vi "Get Status_All Records One.vi"(7 "Timeout (s)":dbl=5.0 caption="Time Target (s)", 8 "error in":errorcluster, 11 "FPGA VI Reference In":refnum<k20>) -> (0 "error out":errorcluster, 2 "Records Done":u32, 3 "FPGA VI Reference Out":refnum<k20>)   [LabVIEW 2011]
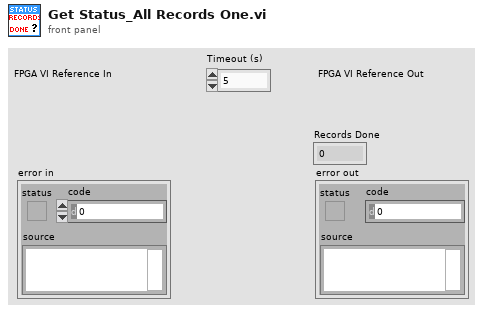
[diagram p1: front panel]
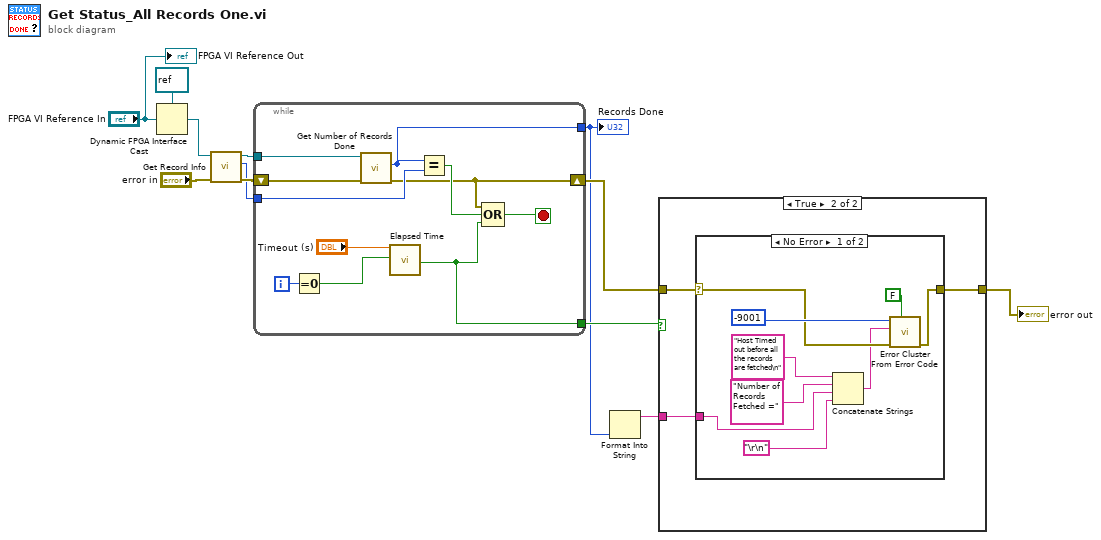
[diagram p0: block diagram]
diagram:
  n1 = Dynamic FPGA Interface Cast(Session In=refnum<k20> refnum ("Type"), Type="FPGA VI Reference In") -> (Session Out=w8:refnum<k20>)
  n2 = call <userlib>:"Get Record Info.vi"("error in"="error in", "FPGA VI Reference In"=w8) -> ("error out"=w12:errorcluster, "Records to Acquire"=w10:u32, "FPGA VI Reference Out"=w11:refnum<k20>)  [unwired: 5 in, 2 out]
  n3 = while {
    tunnel: w11 -> [w21]
    shift-right: [w16] -> w4
    shift-left: w12 -> [w23]
    tunnel: w10 -> [w22]
    tunnel: [w20] -> w2
    tunnel: [w15] -> w5
    i -> [w14]
    stop <- w17 stop-if-true
    n4 = Equal To 0?(x=w14) -> (x = 0?=w13:bool)
    n5 = call <userlib>:"Get Number of Records Done.vi"("error in"=w23, "FPGA VI Reference In"=w21) -> ("error out"=w16:errorcluster, "Records Done"=w20:u32)  [unwired: 7 in, 1 out]
    n6 = call "Elapsed Time"("Time Target (s)"="Timeout (s)", "Reset"=w13) -> ("Time has Elapsed"=w15:bool)  [unwired: 10 in, 7 out]
    n7 = Equal?(x=w20, y=w22) -> (x = y?=w18:bool)
    n8 = Compound Arithmetic op=OR(w16, w18, w15) -> (w17:bool)
  }
  "Records Done" <- w2
  n9 = Format Into String(w2) -> (resulting string=w1:string)  [unwired: 3 in, 1 out]
  n10 = case shown="True" w5 {
    tunnel: w4 -> [w24 w27]
    tunnel: [w24 w26] -> w3
    tunnel: w1 -> [_ w25]
    frame False {
    }
    frame True {
      n11 = case shown="No Error" w27 {
        selector: w27 -> [w34 w37]
        tunnel: [w33 w37] -> w26
        tunnel: w25 -> [w29 _]
        frame No Error {
          n12 = Concatenate Strings("Host Timed out before all the records are fetched\n" ("source"), "Number of Records Fetched =" ("source"), w29, "\r\n") -> (w31:string)
          n13 = call <vilib>:"Error Cluster From Error Code.vi"("show call chain? (False)"=FALSE, "error in (no error)"=w34, "error message (\"\")"=w31, "error code (0)"=-9001 ("code")) -> ("error out"=w33:errorcluster)  [unwired: 5 in]
        }
        frame Error {
        }
      }
    }
  }
  "error out" <- w3
  "FPGA VI Reference Out" <- "FPGA VI Reference In"
